vi "Set Identifier.vi"(1 "Custom ID":string) -> (0 "Example Custom ID out":refnum<class "Example Custom ID.lvclass">)   [LabVIEW 2020, in "serenial.io-ase.example.lvlib" / "Example Custom ID.lvclass"]
uses:
  Example Custom ID.lvclass
  Example Custom ID.lvclass/Example Custom ID.ctl
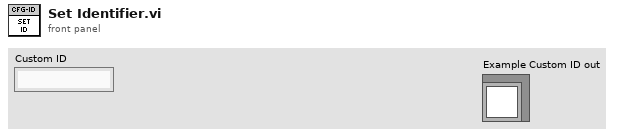
[diagram p1: front panel]
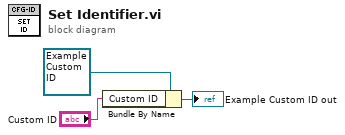
[diagram p0: block diagram]
diagram:
  n1 = Bundle By Name(cluster=refnum<class "Example Custom ID.lvclass"> refnum ("Example Custom ID out"), "Custom ID"="Custom ID") -> (→"Example Custom ID out":refnum<class "Example Custom ID.lvclass">)
